vi "SDG60ConfBurstSplitTrig.vi"() -> ()   [LabVIEW 2018]
panel:
  in  "Trigger Out Mode (0: Off)":u16(ring) items=["Off", "Rise", "Fall"]
  in  "Trigger Source (0: Internal)":i32(ring) items=["Internal", "External", "Manual"]
  in  "Channel (1:Channel 1)":i32(ring)=1 items=["Channel 1"=1, "Channel 2"=2]
  in  "error in (no error)":errorcluster
  out "error out":errorcluster
  in  "VISA resource name":refnum<visa-resource-name>="USB0::0xF4EC::0x1101::SDG6XEBC5R0119::INSTR"
  out "VISA resource name out":refnum<visa-resource-name>
  # "Note: Ext TRG input is the same as output.\nOutput hardwired here to Off all the time!\n\nComplex behaviour:\nTrigger out ignored when gated \nand/or TrigSrc is Ext\nMust be in NCYC,not gated, beforehand\nAux out is 5V\nIf switched from rise to fall, output will\nnot change state immediately"
  # "Burst must be enabled before using this vi\nUse this vi only for triggered mode.\nFor gated mode source is set in burst config\nDon't use this vi when already set to gated mode."
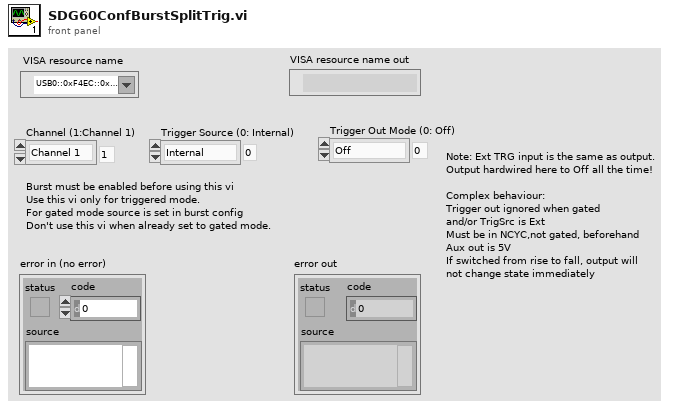
[diagram p1: front panel]
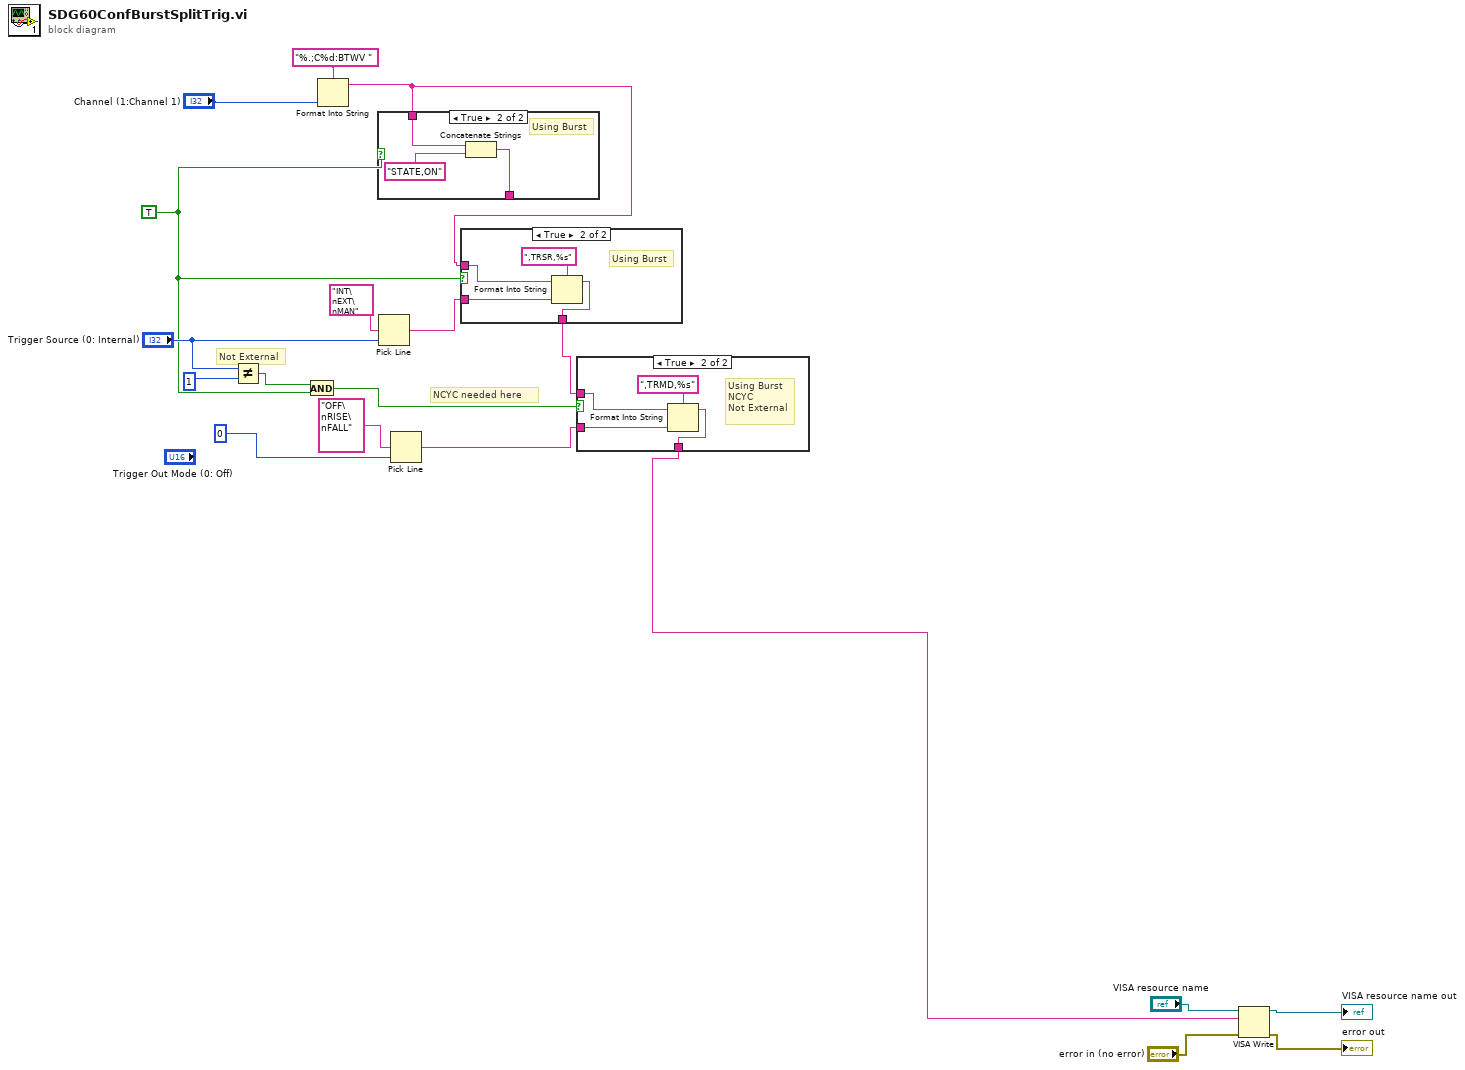
[diagram p0: block diagram]
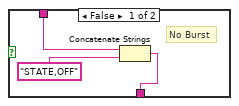
[diagram p4: hidden frame]
diagram:
  w2 = TRUE
  # "NCYC needed here"
  # "Not External"
  n1 = Not Equal?(x="Trigger Source (0: Internal)", y=1) -> (x != y?=w6:bool)
  n2 = And(x=w6, y=w2) -> (x .and. y?=w4:bool)
  n3 = Format Into String(format string="%.;C%d:BTWV ", "Channel (1:Channel 1)") -> (resulting string=w1:string)  [unwired: 2 in, 1 out]
  n4 = case shown="True" w2 {
    tunnel: w1 -> [w22 w25]
    tunnel: [w20 w23] -> _
    frame False {
      # "No Burst"
      n5 = Concatenate Strings(w22, "STATE,OFF") -> (w20:string)
    }
    frame True {
      # "Using Burst"
      n6 = Concatenate Strings(w25, "STATE,ON") -> (w23:string)
    }
  }
  n7 = Pick Line(multi-line string="INT\nEXT\nMAN", line index="Trigger Source (0: Internal)") -> (output string=w13:string)  [unwired: 1 in]
  n8 = Pick Line(multi-line string="OFF\nRISE\nFALL", line index=0) -> (output string=w9:string)  [unwired: 1 in]
  n9 = case shown="True" w2 {
    tunnel: w1 -> [w26 w30]
    tunnel: [w26 w29] -> w11
    tunnel: w13 -> [_ w28]
    frame False {
      # "No Burst"
    }
    frame True {
      # "Using Burst"
      n10 = Format Into String(format string=",TRSR,%s", initial string=w30, w28) -> (resulting string=w29:string)  [unwired: 1 in, 1 out]
    }
  }
  n11 = case shown="True" w4 {
    tunnel: w11 -> [w31 w35]
    tunnel: [w31 w34] -> w5
    tunnel: w9 -> [_ w33]
    frame False {
      # "not using burst or\ngated or external"
    }
    frame True {
      # "Using Burst\nNCYC\nNot External"
      n12 = Format Into String(format string=",TRMD,%s", initial string=w35, w33) -> (resulting string=w34:string)  [unwired: 1 in, 1 out]
    }
  }
  n13 = VISA Write(VISA resource name="VISA resource name", write buffer=w5, error in (no error)="error in (no error)") -> (VISA resource name out=→"VISA resource name out":refnum<visa-resource-name>, error out=→"error out":errorcluster)  [unwired: 1 out]
